vi "Image file metadata dotNET.vi"() -> ()   [LabVIEW 2023]
uses:
  System.Drawing
panel:
  out "PropertyIdList":i32[](array[numeric]) format="%04x"
  in  "EXIF Data list":T1(array[cluster])=[{"ID"=254, "Name"="NewSubfileType", "Notes"="A general indication of the kind of data contained in this subfile."}, {"ID"=255, "Name"="SubfileType", "Notes"="A general indication of the kind of data contained in this subfile."}, {"ID"=256, "Name"="ImageWidth", "Notes"="\"The number of columns in the image, i.e., the number of pixels per row.\""}, {"ID"=257, "Name"="ImageLength", "Notes"="The number of rows of pixels in the image."}, {"ID"=258, "Name"="BitsPerSample", "Notes"="Number of bits per component."}, {"ID"=259, "Name"="Compression", "Notes"="Compression scheme used on the image data."}, {"ID"=262, "Name"="PhotometricInterpretation", "Notes"="The color space of the image data."}, {"ID"=263, "Name"="Threshholding", "Notes"="\"For black and white TIFF files that represent shades of gray, the technique used to convert from gray to black and white pixels.\""}, {"ID"=264, "Name"="CellWidth", "Notes"="The width of the dithering or halftoning matrix used to create a dithered or halftoned bilevel file."}, {"ID"=265, "Name"="CellLength", "Notes"="The length of the dithering or halftoning matrix used to create a dithered or halftoned bilevel file."}, {"ID"=266, "Name"="FillOrder", "Notes"="The logical order of bits within a byte."}, {"ID"=269, "Name"="DocumentName", "Notes"="The name of the document from which this image was scanned."}, {"ID"=270, "Name"="ImageDescription", "Notes"="A string that describes the subject of the image."}, {"ID"=271, "Name"="Make", "Notes"="The scanner manufacturer."}, {"ID"=272, "Name"="Model", "Notes"="The scanner model name or number."}, {"ID"=273, "Name"="StripOffsets", "Notes"="\"For each strip, the byte offset of that strip.\""}, {"ID"=274, "Name"="Orientation", "Notes"="The orientation of the image with respect to the rows and columns."}, {"ID"=277, "Name"="SamplesPerPixel", "Notes"="The number of components per pixel."}, {"ID"=278, "Name"="RowsPerStrip", "Notes"="The number of rows per strip."}, {"ID"=279, "Name"="StripByteCounts", "Notes"="\"For each strip, the number of bytes in the strip after compression.\""}, {"ID"=280, "Name"="MinSampleValue", "Notes"="The minimum component value used."}, {"ID"=281, "Name"="MaxSampleValue", "Notes"="The maximum component value used."}, {"ID"=282, "Name"="XResolution", "Notes"="The number of pixels per ResolutionUnit in the ImageWidth direction."}, {"ID"=283, "Name"="YResolution", "Notes"="The number of pixels per ResolutionUnit in the ImageLength direction."}, {"ID"=284, "Name"="PlanarConfiguration", "Notes"="How the components of each pixel are stored."}, {"ID"=285, "Name"="PageName", "Notes"="The name of the page from which this image was scanned."}, {"ID"=286, "Name"="XPosition", "Notes"="X position of the image."}, {"ID"=287, "Name"="YPosition", "Notes"="Y position of the image."}, {"ID"=288, "Name"="FreeOffsets", "Notes"="\"For each string of contiguous unused bytes in a TIFF file, the byte offset of the string.\""}, {"ID"=289, "Name"="FreeByteCounts", "Notes"="\"For each string of contiguous unused bytes in a TIFF file, the number of bytes in the string.\""}, {"ID"=290, "Name"="GrayResponseUnit", "Notes"="The precision of the information contained in the GrayResponseCurve."}, {"ID"=291, "Name"="GrayResponseCurve", "Notes"="\"For grayscale data, the optical density of each possible pixel value.\""}, {"ID"=292, "Name"="T4Options", "Notes"="Options for Group 3 Fax compression"}, {"ID"=293, "Name"="T6Options", "Notes"="Options for Group 4 Fax compression"}, {"ID"=296, "Name"="ResolutionUnit", "Notes"="The unit of measurement for XResolution and YResolution."}, {"ID"=297, "Name"="PageNumber", "Notes"="The page number of the page from which this image was scanned."}, {"ID"=301, "Name"="TransferFunction", "Notes"="Describes a transfer function for the image in tabular style."}, {"ID"=305, "Name"="Software", "Notes"="Name and version number of the software package(s) used to create the image."}, {"ID"=306, "Name"="DateTime", "Notes"="Date and time of image creation."}, {"ID"=315, "Name"="Artist", "Notes"="Person who created the image."}, {"ID"=316, "Name"="HostComputer", "Notes"="The computer and/or operating system in use at the time of image creation."}, {"ID"=317, "Name"="Predictor", "Notes"="A mathematical operator that is applied to the image data before an encoding scheme is applied."}, {"ID"=318, "Name"="WhitePoint", "Notes"="The chromaticity of the white point of the image."}, {"ID"=319, "Name"="PrimaryChromaticities", "Notes"="The chromaticities of the primaries of the image."}, {"ID"=320, "Name"="ColorMap", "Notes"="A color map for palette color images."}, {"ID"=321, "Name"="HalftoneHints", "Notes"="Conveys to the halftone function the range of gray levels within a colorimetrically-specified image that should retain tonal detail."}, {"ID"=322, "Name"="TileWidth", "Notes"="The tile width in pixels. This is the number of columns in each tile."}, {"ID"=323, "Name"="TileLength", "Notes"="The tile length (height) in pixels. This is the number of rows in each tile."}, {"ID"=324, "Name"="TileOffsets", "Notes"="\"For each tile, the byte offset of that tile, as compressed and stored on disk.\""}, {"ID"=325, "Name"="TileByteCounts", "Notes"="\"For each tile, the number of (compressed) bytes in that tile.\""}, {"ID"=326, "Name"="BadFaxLines", "Notes"="\"Used in the TIFF-F standard, denotes the number of 'bad' scan lines encountered by the facsimile device.\""}, {"ID"=327, "Name"="CleanFaxData", "Notes"="\"Used in the TIFF-F standard, indicates if 'bad' lines encountered during reception are stored in the data, or if 'bad' lines have been replaced by the receiver.\""}, {"ID"=328, "Name"="ConsecutiveBadFaxLines", "Notes"="\"Used in the TIFF-F standard, denotes the maximum number of consecutive 'bad' scanlines received.\""}, {"ID"=330, "Name"="SubIFDs", "Notes"="Offset to child IFDs."}, {"ID"=332, "Name"="InkSet", "Notes"="The set of inks used in a separated (PhotometricInterpretation=5) image."}, {"ID"=333, "Name"="InkNames", "Notes"="The name of each ink used in a separated image."}, {"ID"=334, "Name"="NumberOfInks", "Notes"="The number of inks."}, {"ID"=336, "Name"="DotRange", "Notes"="The component values that correspond to a 0% dot and 100% dot."}, {"ID"=337, "Name"="TargetPrinter", "Notes"="A description of the printing environment for which this separation is intended."}, {"ID"=338, "Name"="ExtraSamples", "Notes"="Description of extra components."}, {"ID"=339, "Name"="SampleFormat", "Notes"="Specifies how to interpret each data sample in a pixel."}, {"ID"=340, "Name"="SMinSampleValue", "Notes"="Specifies the minimum sample value."}, {"ID"=341, "Name"="SMaxSampleValue", "Notes"="Specifies the maximum sample value."}, {"ID"=342, "Name"="TransferRange", "Notes"="Expands the range of the TransferFunction."}, {"ID"=343, "Name"="ClipPath", "Notes"="Mirrors the essentials of PostScript's path creation functionality."}, {"ID"=344, "Name"="XClipPathUnits", "Notes"="\"The number of units that span the width of the image, in terms of integer ClipPath coordinates.\""}, {"ID"=345, "Name"="YClipPathUnits", "Notes"="\"The number of units that span the height of the image, in terms of integer ClipPath coordinates.\""}, {"ID"=346, "Name"="Indexed", "Notes"="Aims to broaden the support for indexed images to include support for any color space."}, {"ID"=347, "Name"="JPEGTables", "Notes"="JPEG quantization and/or Huffman tables."}, {"ID"=351, "Name"="OPIProxy", "Notes"="OPI-related."}, {"ID"=400, "Name"="GlobalParametersIFD", "Notes"="Used in the TIFF-FX standard to point to an IFD containing tags that are globally applicable to the complete TIFF file."}, {"ID"=401, "Name"="ProfileType", "Notes"="\"Used in the TIFF-FX standard, denotes the type of data stored in this file or IFD.\""}, {"ID"=402, "Name"="FaxProfile", "Notes"="\"Used in the TIFF-FX standard, denotes the 'profile' that applies to this file.\""}, {"ID"=403, "Name"="CodingMethods", "Notes"="\"Used in the TIFF-FX standard, indicates which coding methods are used in the file.\""}, {"ID"=404, "Name"="VersionYear", "Notes"="\"Used in the TIFF-FX standard, denotes the year of the standard specified by the FaxProfile field.\""}, {"ID"=405, "Name"="ModeNumber", "Notes"="\"Used in the TIFF-FX standard, denotes the mode of the standard specified by the FaxProfile field.\""}, {"ID"=433, "Name"="Decode", "Notes"="\"Used in the TIFF-F and TIFF-FX standards, holds information about the ITULAB (PhotometricInterpretation = 10) encoding.\""}, {"ID"=434, "Name"="DefaultImageColor", "Notes"="\"Defined in the Mixed Raster Content part of RFC 2301, is the default color needed in areas where no image is available.\""}, {"ID"=512, "Name"="JPEGProc", "Notes"="Old-style JPEG compression field. TechNote2 invalidates this part of the specification."}, {"ID"=513, "Name"="JPEGInterchangeFormat", "Notes"="Old-style JPEG compression field. TechNote2 invalidates this part of the specification."}, {"ID"=514, "Name"="JPEGInterchangeFormatLength", "Notes"="Old-style JPEG compression field. TechNote2 invalidates this part of the specification."}, {"ID"=515, "Name"="JPEGRestartInterval", "Notes"="Old-style JPEG compression field. TechNote2 invalidates this part of the specification."}, {"ID"=517, "Name"="JPEGLosslessPredictors", "Notes"="Old-style JPEG compression field. TechNote2 invalidates this part of the specification."}, {"ID"=518, "Name"="JPEGPointTransforms", "Notes"="Old-style JPEG compression field. TechNote2 invalidates this part of the specification."}, {"ID"=519, "Name"="JPEGQTables", "Notes"="Old-style JPEG compression field. TechNote2 invalidates this part of the specification."}, {"ID"=520, "Name"="JPEGDCTables", "Notes"="Old-style JPEG compression field. TechNote2 invalidates this part of the specification."}, {"ID"=521, "Name"="JPEGACTables", "Notes"="Old-style JPEG compression field. TechNote2 invalidates this part of the specification."}, {"ID"=529, "Name"="YCbCrCoefficients", "Notes"="The transformation from RGB to YCbCr image data."}, {"ID"=530, "Name"="YCbCrSubSampling", "Notes"="Specifies the subsampling factors used for the chrominance components of a YCbCr image."}, {"ID"=531, "Name"="YCbCrPositioning", "Notes"="Specifies the positioning of subsampled chrominance components relative to luminance samples."}, {"ID"=532, "Name"="ReferenceBlackWhite", "Notes"="Specifies a pair of headroom and footroom image data values (codes) for each pixel component."}, {"ID"=559, "Name"="StripRowCounts", "Notes"="\"Defined in the Mixed Raster Content part of RFC 2301, used to replace RowsPerStrip for IFDs with variable-sized strips.\""}, {"ID"=700, "Name"="XMP", "Notes"="XML packet containing XMP metadata"}, {"ID"=32781, "Name"="ImageID", "Notes"="OPI-related."}, {"ID"=32932, "Name"="Wang Annotation", "Notes"="\"Annotation data, as used in 'Imaging for Windows'.\""}, {"ID"=33432, "Name"="Copyright", "Notes"="Copyright notice."}, {"ID"=33434, "Name"="ExposureTime", "Notes"="\"Exposure time, given in seconds.\""}, {"ID"=33437, "Name"="FNumber", "Notes"="The F number."}, {"ID"=33445, "Name"="MD FileTag", "Notes"="Specifies the pixel data format encoding in the Molecular Dynamics GEL file format."}, {"ID"=33446, "Name"="MD ScalePixel", "Notes"="Specifies a scale factor in the Molecular Dynamics GEL file format."}, {"ID"=33447, "Name"="MD ColorTable", "Notes"="Used to specify the conversion from 16bit to 8bit in the Molecular Dynamics GEL file format."}, {"ID"=33448, "Name"="MD LabName", "Notes"="\"Name of the lab that scanned this file, as used in the Molecular Dynamics GEL file format.\""}, {"ID"=33449, "Name"="MD SampleInfo", "Notes"="\"Information about the sample, as used in the Molecular Dynamics GEL file format.\""}, {"ID"=33450, "Name"="MD PrepDate", "Notes"="\"Date the sample was prepared, as used in the Molecular Dynamics GEL file format.\""}, {"ID"=33451, "Name"="MD PrepTime", "Notes"="\"Time the sample was prepared, as used in the Molecular Dynamics GEL file format.\""}, {"ID"=33452, "Name"="MD FileUnits", "Notes"="\"Units for data in this file, as used in the Molecular Dynamics GEL file format.\""}, {"ID"=33550, "Name"="ModelPixelScaleTag", "Notes"="Used in interchangeable GeoTIFF files."}, {"ID"=33723, "Name"="IPTC", "Notes"="IPTC (International Press Telecommunications Council) metadata."}, {"ID"=33918, "Name"="INGR Packet Data Tag", "Notes"="Intergraph Application specific storage."}, {"ID"=33919, "Name"="INGR Flag Registers", "Notes"="Intergraph Application specific flags."}, {"ID"=33920, "Name"="IrasB Transformation Matrix", "Notes"="\"Originally part of Intergraph's GeoTIFF tags, but likely understood by IrasB only.\""}, {"ID"=33922, "Name"="ModelTiepointTag", "Notes"="\"Originally part of Intergraph's GeoTIFF tags, but now used in interchangeable GeoTIFF files.\""}, {"ID"=34264, "Name"="ModelTransformationTag", "Notes"="Used in interchangeable GeoTIFF files."}, {"ID"=34377, "Name"="Photoshop", "Notes"="Collection of Photoshop 'Image Resource Blocks'."}, {"ID"=34665, "Name"="Exif IFD", "Notes"="A pointer to the Exif IFD."}, {"ID"=34675, "Name"="ICC Profile", "Notes"="ICC profile data."}, {"ID"=34732, "Name"="ImageLayer", "Notes"="\"Defined in the Mixed Raster Content part of RFC 2301, used to denote the particular function of this Image in the mixed raster scheme.\""}, {"ID"=34735, "Name"="GeoKeyDirectoryTag", "Notes"="Used in interchangeable GeoTIFF files."}, {"ID"=34736, "Name"="GeoDoubleParamsTag", "Notes"="Used in interchangeable GeoTIFF files."}, {"ID"=34737, "Name"="GeoAsciiParamsTag", "Notes"="Used in interchangeable GeoTIFF files."}, {"ID"=34850, "Name"="ExposureProgram", "Notes"="The class of the program used by the camera to set exposure when the picture is taken."}, {"ID"=34852, "Name"="SpectralSensitivity", "Notes"="Indicates the spectral sensitivity of each channel of the camera used."}, {"ID"=34853, "Name"="GPS IFD", "Notes"="A pointer to the Exif-related GPS Info IFD."}, {"ID"=34855, "Name"="ISOSpeedRatings", "Notes"="Indicates the ISO Speed and ISO Latitude of the camera or input device as specified in ISO 12232."}, {"ID"=34856, "Name"="OECF", "Notes"="Indicates the Opto-Electric Conversion Function (OECF) specified in ISO 14524."}, {"ID"=34908, "Name"="HylaFAX FaxRecvParams", "Notes"="Used by HylaFAX."}, {"ID"=34909, "Name"="HylaFAX FaxSubAddress", "Notes"="Used by HylaFAX."}, {"ID"=34910, "Name"="HylaFAX FaxRecvTime", "Notes"="Used by HylaFAX."}, {"ID"=36864, "Name"="ExifVersion", "Notes"="The version of the supported Exif standard."}, {"ID"=36867, "Name"="DateTimeOriginal", "Notes"="The date and time when the original image data was generated."}, {"ID"=36868, "Name"="DateTimeDigitized", "Notes"="The date and time when the image was stored as digital data."}, {"ID"=37121, "Name"="ComponentsConfiguration", "Notes"="Specific to compressed data; specifies the channels and complements PhotometricInterpretation"}, {"ID"=37122, "Name"="CompressedBitsPerPixel", "Notes"="Specific to compressed data; states the compressed bits per pixel."}, {"ID"=37377, "Name"="ShutterSpeedValue", "Notes"="Shutter speed."}, {"ID"=37378, "Name"="ApertureValue", "Notes"="The lens aperture."}, {"ID"=37379, "Name"="BrightnessValue", "Notes"="The value of brightness."}, {"ID"=37380, "Name"="ExposureBiasValue", "Notes"="The exposure bias."}, {"ID"=37381, "Name"="MaxApertureValue", "Notes"="The smallest F number of the lens."}, {"ID"=37382, "Name"="SubjectDistance", "Notes"="\"The distance to the subject, given in meters.\""}, {"ID"=37383, "Name"="MeteringMode", "Notes"="The metering mode."}, {"ID"=37384, "Name"="LightSource", "Notes"="The kind of light source."}, {"ID"=37385, "Name"="Flash", "Notes"="Indicates the status of flash when the image was shot."}, {"ID"=37386, "Name"="FocalLength", "Notes"="\"The actual focal length of the lens, in mm.\""}, {"ID"=37396, "Name"="SubjectArea", "Notes"="Indicates the location and area of the main subject in the overall scene."}, {"ID"=37500, "Name"="MakerNote", "Notes"="Manufacturer specific information."}, {"ID"=37510, "Name"="UserComment", "Notes"="Keywords or comments on the image; complements ImageDescription."}, {"ID"=37520, "Name"="SubsecTime", "Notes"="A tag used to record fractions of seconds for the DateTime tag."}, {"ID"=37521, "Name"="SubsecTimeOriginal", "Notes"="A tag used to record fractions of seconds for the DateTimeOriginal tag."}, {"ID"=37522, "Name"="SubsecTimeDigitized", "Notes"="A tag used to record fractions of seconds for the DateTimeDigitized tag."}, {"ID"=37724, "Name"="ImageSourceData", "Notes"="Used by Adobe Photoshop."}, {"ID"=40960, "Name"="FlashpixVersion", "Notes"="The Flashpix format version supported by a FPXR file."}, {"ID"=40961, "Name"="ColorSpace", "Notes"="The color space information tag is always recorded as the color space specifier."}, {"ID"=40962, "Name"="PixelXDimension", "Notes"="Specific to compressed data; the valid width of the meaningful image."}, {"ID"=40963, "Name"="PixelYDimension", "Notes"="Specific to compressed data; the valid height of the meaningful image."}, {"ID"=40964, "Name"="RelatedSoundFile", "Notes"="Used to record the name of an audio file related to the image data."}, {"ID"=40965, "Name"="Interoperability IFD", "Notes"="A pointer to the Exif-related Interoperability IFD."}, {"ID"=41483, "Name"="FlashEnergy", "Notes"="\"Indicates the strobe energy at the time the image is captured, as measured in Beam Candle Power Seconds\""}, {"ID"=41484, "Name"="SpatialFrequencyResponse", "Notes"="\"Records the camera or input device spatial frequency table and SFR values in the direction of image width, image height, and diagonal direction, as specified in ISO 12233.\""}, {"ID"=41486, "Name"="FocalPlaneXResolution", "Notes"="Indicates the number of pixels in the image width (X) direction per FocalPlaneResolutionUnit on the camera focal plane."}, {"ID"=41487, "Name"="FocalPlaneYResolution", "Notes"="Indicates the number of pixels in the image height (Y) direction per FocalPlaneResolutionUnit on the camera focal plane."}, {"ID"=41488, "Name"="FocalPlaneResolutionUnit", "Notes"="Indicates the unit for measuring FocalPlaneXResolution and FocalPlaneYResolution."}, {"ID"=41492, "Name"="SubjectLocation", "Notes"="Indicates the location of the main subject in the scene."}, {"ID"=41493, "Name"="ExposureIndex", "Notes"="Indicates the exposure index selected on the camera or input device at the time the image is captured."}, {"ID"=41495, "Name"="SensingMethod", "Notes"="Indicates the image sensor type on the camera or input device."}, {"ID"=41728, "Name"="FileSource", "Notes"="Indicates the image source."}, {"ID"=41729, "Name"="SceneType", "Notes"="Indicates the type of scene."}, {"ID"=41730, "Name"="CFAPattern", "Notes"="Indicates the color filter array (CFA) geometric pattern of the image sensor when a one-chip color area sensor is used."}, {"ID"=41985, "Name"="CustomRendered", "Notes"="\"Indicates the use of special processing on image data, such as rendering geared to output.\""}, {"ID"=41986, "Name"="ExposureMode", "Notes"="Indicates the exposure mode set when the image was shot."}, {"ID"=41987, "Name"="WhiteBalance", "Notes"="Indicates the white balance mode set when the image was shot."}, {"ID"=41988, "Name"="DigitalZoomRatio", "Notes"="Indicates the digital zoom ratio when the image was shot."}, {"ID"=41989, "Name"="FocalLengthIn35mmFilm", "Notes"="\"Indicates the equivalent focal length assuming a 35mm film camera, in mm.\""}, {"ID"=41990, "Name"="SceneCaptureType", "Notes"="Indicates the type of scene that was shot."}, {"ID"=41991, "Name"="GainControl", "Notes"="Indicates the degree of overall image gain adjustment."}, {"ID"=41992, "Name"="Contrast", "Notes"="Indicates the direction of contrast processing applied by the camera when the image was shot."}, {"ID"=41993, "Name"="Saturation", "Notes"="Indicates the direction of saturation processing applied by the camera when the image was shot."}, {"ID"=41994, "Name"="Sharpness", "Notes"="Indicates the direction of sharpness processing applied by the camera when the image was shot."}, {"ID"=41995, "Name"="DeviceSettingDescription", "Notes"="This tag indicates information on the picture-taking conditions of a particular camera model."}, {"ID"=41996, "Name"="SubjectDistanceRange", "Notes"="Indicates the distance to the subject."}, {"ID"=42016, "Name"="ImageUniqueID", "Notes"="Indicates an identifier assigned uniquely to each image."}, {"ID"=42112, "Name"="GDAL_METADATA", "Notes"="\"Used by the GDAL library, holds an XML list of name=value 'metadata' values about the image as a whole, and about specific samples.\""}, {"ID"=42113, "Name"="GDAL_NODATA", "Notes"="\"Used by the GDAL library, contains an ASCII encoded nodata or background pixel value.\""}, {"ID"=50215, "Name"="Oce Scanjob Description", "Notes"="Used in the Oce scanning process."}, {"ID"=50216, "Name"="Oce Application Selector", "Notes"="Used in the Oce scanning process."}, {"ID"=50217, "Name"="Oce Identification Number", "Notes"="Used in the Oce scanning process."}, {"ID"=50218, "Name"="Oce ImageLogic Characteristics", "Notes"="Used in the Oce scanning process."}, {"ID"=50706, "Name"="DNGVersion", "Notes"="Used in IFD 0 of DNG files."}, {"ID"=50707, "Name"="DNGBackwardVersion", "Notes"="Used in IFD 0 of DNG files."}, {"ID"=50708, "Name"="UniqueCameraModel", "Notes"="Used in IFD 0 of DNG files."}, {"ID"=50709, "Name"="LocalizedCameraModel", "Notes"="Used in IFD 0 of DNG files."}, {"ID"=50710, "Name"="CFAPlaneColor", "Notes"="Used in Raw IFD of DNG files."}, {"ID"=50711, "Name"="CFALayout", "Notes"="Used in Raw IFD of DNG files."}, {"ID"=50712, "Name"="LinearizationTable", "Notes"="Used in Raw IFD of DNG files."}, {"ID"=50713, "Name"="BlackLevelRepeatDim", "Notes"="Used in Raw IFD of DNG files."}, {"ID"=50714, "Name"="BlackLevel", "Notes"="Used in Raw IFD of DNG files."}, {"ID"=50715, "Name"="BlackLevelDeltaH", "Notes"="Used in Raw IFD of DNG files."}, {"ID"=50716, "Name"="BlackLevelDeltaV", "Notes"="Used in Raw IFD of DNG files."}, {"ID"=50717, "Name"="WhiteLevel", "Notes"="Used in Raw IFD of DNG files."}, {"ID"=50718, "Name"="DefaultScale", "Notes"="Used in Raw IFD of DNG files."}, {"ID"=50719, "Name"="DefaultCropOrigin", "Notes"="Used in Raw IFD of DNG files."}, {"ID"=50720, "Name"="DefaultCropSize", "Notes"="Used in Raw IFD of DNG files."}, {"ID"=50721, "Name"="ColorMatrix1", "Notes"="Used in IFD 0 of DNG files."}, {"ID"=50722, "Name"="ColorMatrix2", "Notes"="Used in IFD 0 of DNG files."}, {"ID"=50723, "Name"="CameraCalibration1", "Notes"="Used in IFD 0 of DNG files."}, {"ID"=50724, "Name"="CameraCalibration2", "Notes"="Used in IFD 0 of DNG files."}, {"ID"=50725, "Name"="ReductionMatrix1", "Notes"="Used in IFD 0 of DNG files."}, {"ID"=50726, "Name"="ReductionMatrix2", "Notes"="Used in IFD 0 of DNG files."}, {"ID"=50727, "Name"="AnalogBalance", "Notes"="Used in IFD 0 of DNG files."}, {"ID"=50728, "Name"="AsShotNeutral", "Notes"="Used in IFD 0 of DNG files."}, {"ID"=50729, "Name"="AsShotWhiteXY", "Notes"="Used in IFD 0 of DNG files."}, {"ID"=50730, "Name"="BaselineExposure", "Notes"="Used in IFD 0 of DNG files."}, {"ID"=50731, "Name"="BaselineNoise", "Notes"="Used in IFD 0 of DNG files."}, {"ID"=50732, "Name"="BaselineSharpness", "Notes"="Used in IFD 0 of DNG files."}, {"ID"=50733, "Name"="BayerGreenSplit", "Notes"="Used in Raw IFD of DNG files."}, {"ID"=50734, "Name"="LinearResponseLimit", "Notes"="Used in IFD 0 of DNG files."}, {"ID"=50735, "Name"="CameraSerialNumber", "Notes"="Used in IFD 0 of DNG files."}, {"ID"=50736, "Name"="LensInfo", "Notes"="Used in IFD 0 of DNG files."}, {"ID"=50737, "Name"="ChromaBlurRadius", "Notes"="Used in Raw IFD of DNG files."}, {"ID"=50738, "Name"="AntiAliasStrength", "Notes"="Used in Raw IFD of DNG files."}, {"ID"=50740, "Name"="DNGPrivateData", "Notes"="Used in IFD 0 of DNG files."}, {"ID"=50741, "Name"="MakerNoteSafety", "Notes"="Used in IFD 0 of DNG files."}, {"ID"=50778, "Name"="CalibrationIlluminant1", "Notes"="Used in IFD 0 of DNG files."}, {"ID"=50779, "Name"="CalibrationIlluminant2", "Notes"="Used in IFD 0 of DNG files."}, {"ID"=50780, "Name"="BestQualityScale", "Notes"="Used in Raw IFD of DNG files."}, {"ID"=50784, "Name"="Alias Layer Metadata", "Notes"="Alias Sketchbook Pro layer usage description."}]
  in  "fileName":path=path "D:/My VIs/rename test/2008-05-21 (1).jpg"
  out "Image file attributes":T2(array[cluster])
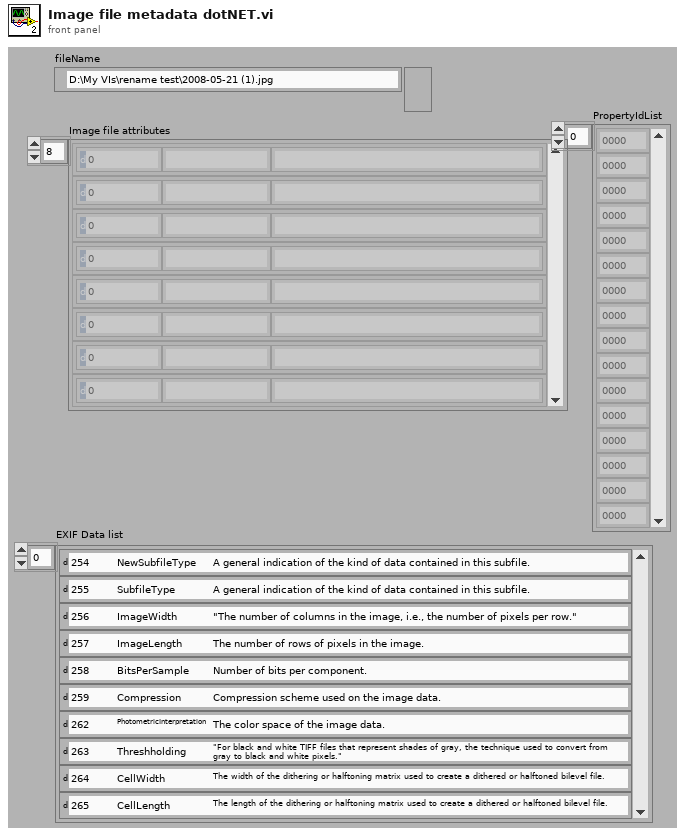
[diagram p1: front panel]
types:
  T1 = cluster{"ID":i32, "Name":string, "Notes":string}[]
  T2 = cluster{"Id":i32, "Name":string, "value":string}[]
  T3 = cluster{"Id":i32, "Name":string, "string":string}
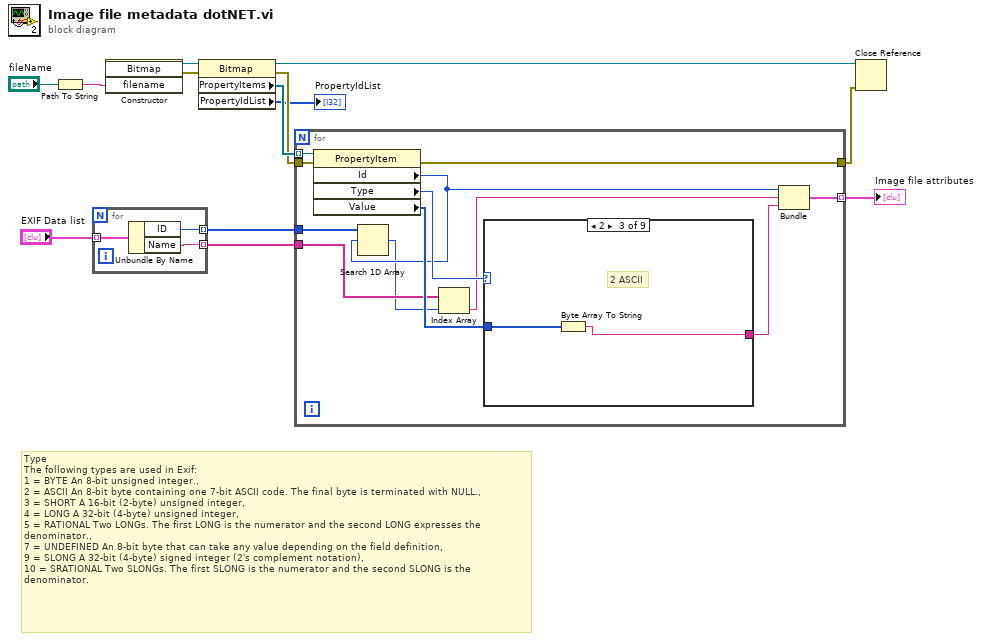
[diagram p0: block diagram]
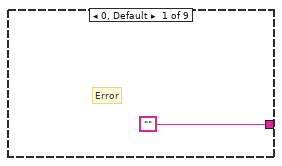
[diagram p2: hidden frame]
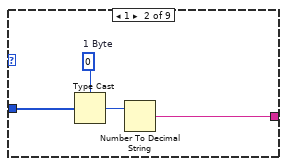
[diagram p3: hidden frame]
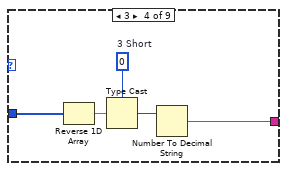
[diagram p4: hidden frame]
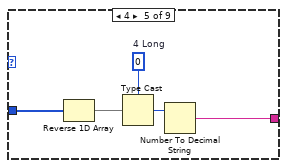
[diagram p5: hidden frame]
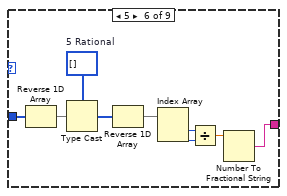
[diagram p6: hidden frame]
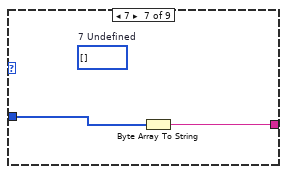
[diagram p7: hidden frame]
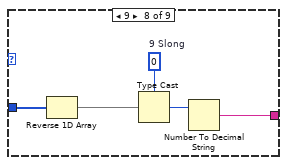
[diagram p8: hidden frame]
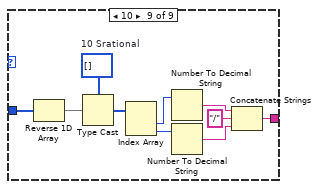
[diagram p9: hidden frame]
diagram:
  # "Type\nThe following types are used in Exif:\n1 = BYTE An 8-bit unsigned integer.,\n2 = ASCII An 8-bit byte containing one 7-bit ASCII code. The final byte is terminated with NULL.,\n3 = SHORT A 16-bit (2-byte) unsigned integer,\n4 = LONG A 32-bit (4-byte) unsigned integer,\n5 = RATIONAL Two LONGs. The first LONG is the numerator and the second LONG expresses the\ndenominator.,\n7 = UNDEFINED An 8-bit byte that can take any value depending on the field definition,\n9 = SLONG A 32-bit (4-byte) signed integer (2's complement notation),\n10 = SRATIONAL Two SLONGs. The first SLONG is the numerator and the second SLONG is the\ndenominator."
  n1 = Path To String(path="fileName") -> (string=w6:string)
  n2 = for {
    tunnel: "EXIF Data list" -> [w16] mode=indexing
    tunnel: [w15] -> w8 mode=indexing
    tunnel: [w14] -> w7 mode=indexing
    n3 = Unbundle By Name(w16) -> ("ID"=w15:i32, "Name"=w14:string)
  }
  n4 = constructor class="Bitmap"("filename"=w6) -> (reference out=w12:refnum<k24>, error out=w5:errorcluster)  [unwired: 3 in, 2 out]
  n5 = property class="Bitmap"(reference=w12, error in=w5) -> (reference out=w1:refnum<k24>, error out=w4:errorcluster, "PropertyItems"=w11:refnum<k24>[], "PropertyIdList"=→"PropertyIdList":i32[])
  n6 = for {
    tunnel: w11 -> [w28] mode=indexing
    tunnel: [w27] -> w10
    tunnel: [w26] -> w9 mode=indexing
    tunnel: w8 -> [w21]
    tunnel: w7 -> [w19]
    tunnel: w4 -> [w25]
    n7 = property class="PropertyItem"(reference=w28, error in=w25) -> (error out=w27:errorcluster, "Id"=w20:i32, "Type"=w22:i16, "Value"=w24:u8[])  [unwired: 1 out]
    n8 = Search 1D Array(1D array=w21, element=w20) -> (index of element=w18:i32)  [unwired: 1 in]
    n9 = Index Array(array=w19, index=w18) -> (element=w17:string)
    n10 = case shown="2" w22 {
      tunnel: w24 -> [_ w33 w35 w40 w45 w54 w56 w61 w71]
      tunnel: ["" w30 w34 w37 w42 w48 w55 w59 w65] -> w23
      frame 0, Default {
        # "Error"
      }
      frame 1 {
        w32 = u8 0  # 1 Byte
        n11 = Type Cast(type=w32, x=w33) -> (*(type *) &x=w31:u8)
        n12 = Number To Decimal String(number=w31) -> (decimal integer string=w30:string)  [unwired: 1 in]
      }
      frame 2 {
        # "2 ASCII"
        n13 = Byte Array To String(unsigned byte array=w35) -> (string=w34:string)
      }
      frame 3 {
        w38 = u16 0  # 3 Short
        n14 = Reverse 1D Array(array=w40) -> (reversed array=w36:u8[])
        n15 = Type Cast(type=w38, x=w36) -> (*(type *) &x=w39:u16)
        n16 = Number To Decimal String(number=w39) -> (decimal integer string=w37:string)  [unwired: 1 in]
      }
      frame 4 {
        w43 = u32 0  # 4 Long
        n17 = Reverse 1D Array(array=w45) -> (reversed array=w41:u8[])
        n18 = Type Cast(type=w43, x=w41) -> (*(type *) &x=w44:u32)
        n19 = Number To Decimal String(number=w44) -> (decimal integer string=w42:string)  [unwired: 1 in]
      }
      frame 5 {
        w53 = u32[] []  # 5 Rational
        n20 = Reverse 1D Array(array=w54) -> (reversed array=w47:u8[])
        n21 = Type Cast(type=w53, x=w47) -> (*(type *) &x=w52:u32[])
        n22 = Reverse 1D Array(array=w52) -> (reversed array=w46:u32[])
        n23 = Index Array(array=w46) -> (element #1=w51:u32, element #2=w50:u32)  [unwired: 2 in]
        n24 = Divide(x=w51, y=w50) -> (x/y=w49:dbl)
        n25 = Number To Fractional String(number=w49) -> (F-format string=w48:string)  [unwired: 3 in]
      }
      frame 7 {
        (unwired) u8[] []  # 7 Undefined
        n26 = Byte Array To String(unsigned byte array=w56) -> (string=w55:string)
      }
      frame 9 {
        w58 = 0  # 9 Slong
        n27 = Reverse 1D Array(array=w61) -> (reversed array=w57:u8[])
        n28 = Type Cast(type=w58, x=w57) -> (*(type *) &x=w60:i32)
        n29 = Number To Decimal String(number=w60) -> (decimal integer string=w59:string)  [unwired: 1 in]
      }
      frame 10 {
        w63 = i32[] []  # 10 Srational
        n30 = Reverse 1D Array(array=w71) -> (reversed array=w62:u8[])
        n31 = Type Cast(type=w63, x=w62) -> (*(type *) &x=w70:i32[])
        n32 = Index Array(array=w70) -> (element #1=w68:i32, element #2=w69:i32)  [unwired: 2 in]
        n33 = Number To Decimal String(number=w68) -> (decimal integer string=w67:string)  [unwired: 1 in]
        n34 = Number To Decimal String(number=w69) -> (decimal integer string=w66:string)  [unwired: 1 in]
        n35 = Concatenate Strings(w67, "/" ("string"), w66) -> (w65:string)
      }
    }
    n36 = Bundle("Id"=w20, "Name"=w17, "string"=w23) -> (w26:T3)  [unwired: 1 in]
  }
  "Image file attributes" <- w9
  n37 = Close Reference(reference=w1, error in (no error)=w10) -> ()  [unwired: 1 out]
